vi "parse_PolynomialTrajectory.vi"(4 "error in":errorcluster, 7 "msg in":string) -> (0 "error out":errorcluster, 2 "Trajectory":T1, 3 "msg out":string)   [LabVIEW 2018]
doc: "Parses a message into an acceleration"
uses:
  Google_Drive/Labview/Robot 3/Typedefs/Polynomial Trajectory typedef.ctl
  Google_Drive/Labview/Robot 3/Typedefs/Polynomial Segment typedef.ctl
  <userlib>/ROS for LabVIEW Software/ROS/MessageParsing/polynomial_msgs/subs/parse_PolynomialSegment_array.vi
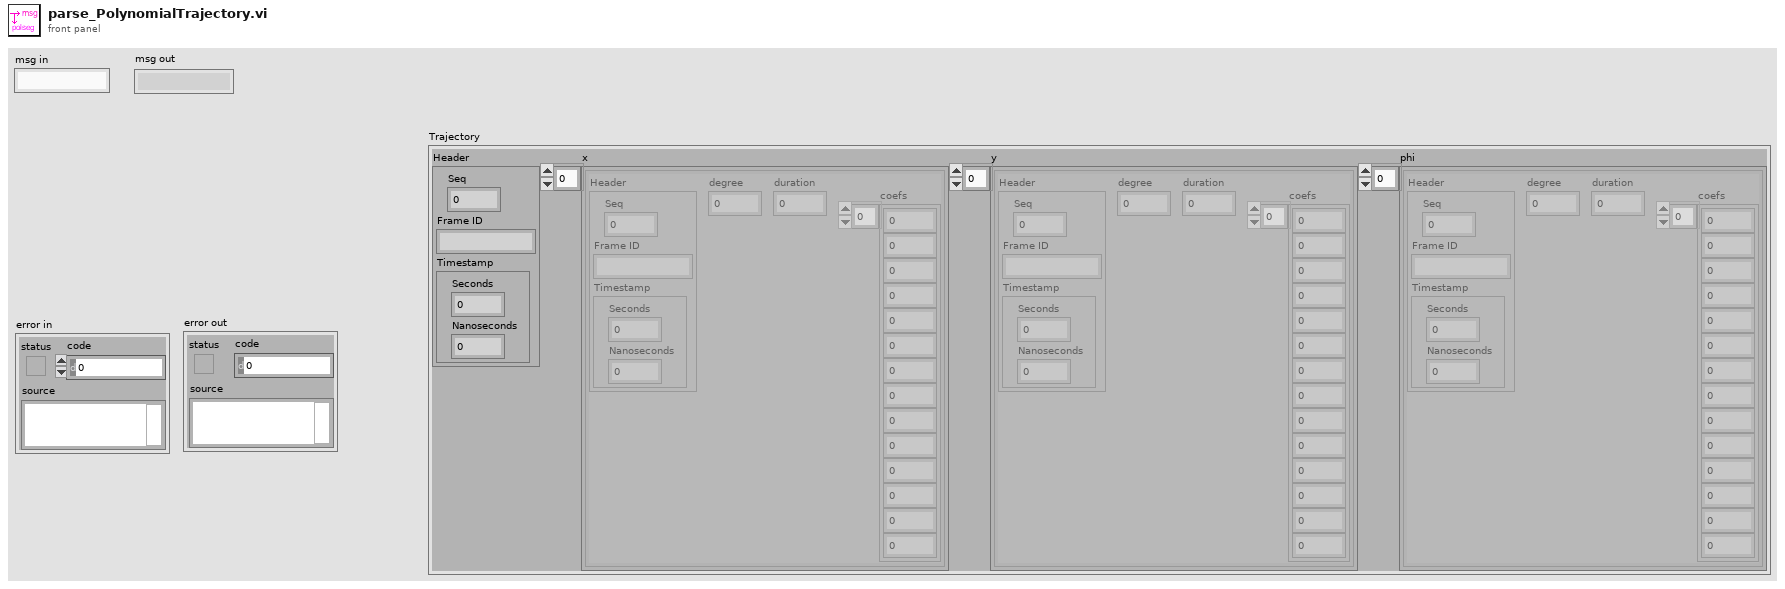
[diagram p1: front panel]
types:
  T1 = typedef "Polynomial Trajectory typedef.ctl" = cluster{"Header":cluster{"Seq":u32, "Frame ID":string, "Timestamp":cluster{"Seconds":i32, "Nanoseconds":i32}}, "x":T2[], "y":T2[], "phi":T2[]}
  T2 = typedef "Polynomial Segment typedef.ctl" = cluster{"Header":cluster{"Seq":u32, "Frame ID":string, "Timestamp":cluster{"Seconds":i32, "Nanoseconds":i32}}, "degree":i32, "duration":dbl, "coefs":dbl[]}
  T3 = cluster{"Seq":u32, "Frame ID":string, "Timestamp":cluster{"Seconds":i32, "Nanoseconds":i32}}
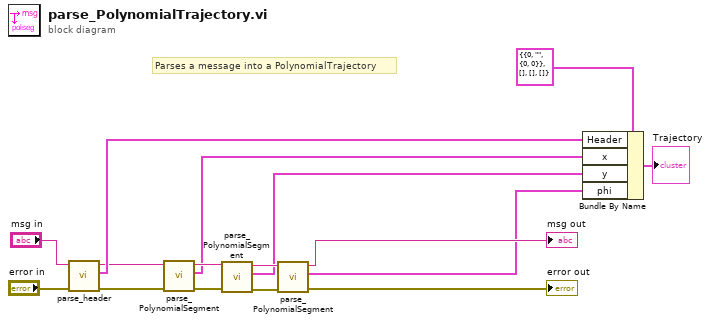
[diagram p0: block diagram]
diagram:
  # "Parses a message into a PolynomialTrajectory"
  n1 = call <userlib>:"parse_header.vi"("error in"="error in", "msg in"="msg in") -> ("error out"=w12:errorcluster, "Header"=w14:T3, "msg out"=w13:string)  [unwired: 3 in]
  n2 = call-poly <userlib>:"parse_PolynomialSegment.vi"("error in"=w12, "msg in"=w13) -> ("error out"=w10:errorcluster, "Polynomial Segment"=w5:T2[], "msg out"=w11:string)  [unwired: 3 in]
  n3 = call-poly <userlib>:"parse_PolynomialSegment.vi"("error in"=w10, "msg in"=w11) -> ("error out"=w8:errorcluster, "Polynomial Segment"=w4:T2[], "msg out"=w9:string)  [unwired: 3 in]
  n4 = call-poly <userlib>:"parse_PolynomialSegment.vi"("error in"=w8, "msg in"=w9) -> ("error out"=→"error out":errorcluster, "Polynomial Segment"=w3:T2[], "msg out"=→"msg out":string)  [unwired: 3 in]
  n5 = Bundle By Name(cluster=T1 {"Header"={"Seq"=0, "Frame ID"="", "Timestamp"={"Seconds"=0, "Nanoseconds"=0}}, "x"=[], "y"=[], "phi"=[]} ("Trajectory"), "Header"=w14, "x"=w5, "y"=w4, "phi"=w3) -> (→"Trajectory":T1)
